vi "Find_Mid_Value.vi"() -> ()   [LabVIEW 2020]
uses:
  <vilib>/DAQmx/read.llb/DAQmx Read (Analog DBL 1Chan 1Samp).vi
  <vilib>/Analysis/baseanly.llb/Mean (DBL).vi
  <vilib>/DAQmx/create/channels.llb/DAQmx Create Channel (AI-Voltage-Basic).vi
  <vilib>/DAQmx/configure/timing.llb/DAQmx Timing (Sample Clock).vi
  <vilib>/DAQmx/miscellaneous.llb/DAQmx Fill In Error Info.vi
  <vilib>/Analysis/NI_AALBase.lvlib
panel:
  out "mean":dbl format="%0.2f"
  out "Final Array":dbl[][](array[numeric])
  out "Initialized Array":dbl[][](array[numeric])
  out "Temperature Array":dbl[][](array[numeric])
  out "error out":errorcluster
  in  "Columns":u8
  in  "Rows":u8
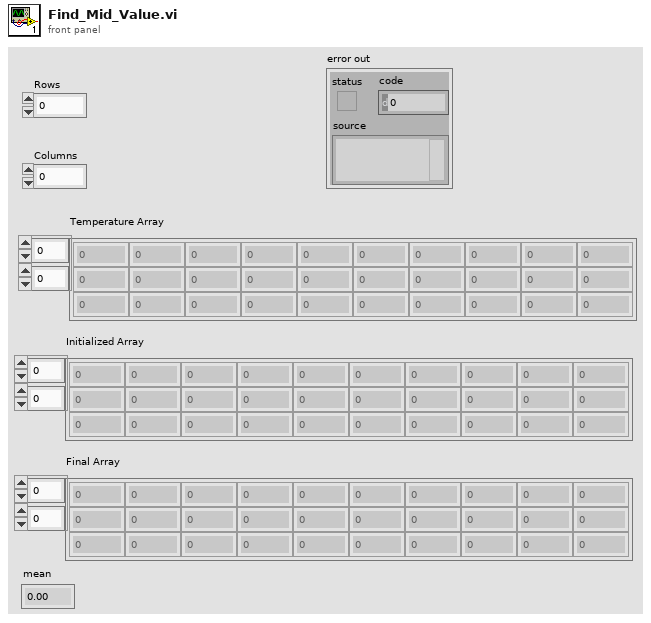
[diagram p1: front panel]
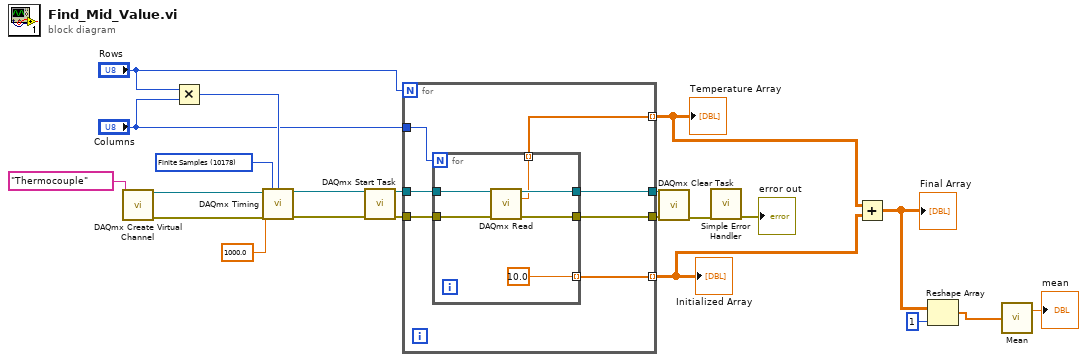
[diagram p0: block diagram]
diagram:
  w18 = 10178 items=["Finite Samples"=10178, "Continuous Samples"=10123, "Hardware Timed Single Point"=12522] ("sample mode")
  n1 = call-poly <vilib>:"DAQmx Create Virtual Channel.vi"("physical channels"=tag "Thermocouple") -> ("task out"=w20:refnum<k21>, "error out"=w21:errorcluster)  [unwired: 13 in]
  n2 = Multiply(x="Rows", y="Columns") -> (x*y=w17:u8)
  n3 = call-poly <vilib>:"DAQmx Timing.vi"("task/channels in"=w20, "sample mode"=w18, "samples per channel"=w17, "rate"=1000.0, "error in"=w21) -> ("task out"=w16:refnum<k21>, "error out"=w15:errorcluster)  [unwired: 9 in]
  n4 = call <vilib>:"DAQmx Start Task.vi"("task/channels in"=w16, "error in"=w15) -> ("task out"=w13:refnum<k21>, "error out"=w14:errorcluster)  [unwired: 12 in]
  n5 = for {
    N: "Rows" -> [_]
    tunnel: "Columns" -> [w25]
    tunnel: w13 -> [w28]
    tunnel: [w27] -> w12
    tunnel: w14 -> [w29]
    tunnel: [w26] -> w11
    tunnel: [w24] -> w6 mode=indexing
    tunnel: [w23] -> w5 mode=indexing
    n6 = for {
      N: w25 -> [_]
      tunnel: w28 -> [w34]
      tunnel: [w33] -> w27
      tunnel: w29 -> [w35]
      tunnel: [w32] -> w26
      tunnel: [w31] -> w24 mode=indexing
      tunnel: [10.0] -> w23 mode=indexing
      n7 = call-poly <vilib>:"DAQmx Read.vi"("task/channels in"=w34, "error in"=w35) -> ("task out"=w33:refnum<k21>, "data"=w31:dbl, "error out"=w32:errorcluster)  [unwired: 11 in]
    }
  }
  "Temperature Array" <- w6
  "Initialized Array" <- w5
  n8 = call <vilib>:"DAQmx Clear Task.vi"("task in"=w12, "error in"=w11) -> ("error out"=w10:errorcluster)  [unwired: 13 in]
  n9 = call <vilib>:"Simple Error Handler.vi"("error in (no error)"=w10) -> ("error out"=→"error out":errorcluster)  [unwired: 4 in, 4 out]
  n10 = Add(x=w6, y=w5) -> (x+y=w3:dbl[][])
  "Final Array" <- w3
  n11 = Reshape Array(w3, 1 ("dimension size")) -> (w1:dbl[])
  n12 = call-poly <vilib>:"Mean.vi"("X"=w1) -> ("mean"=→"mean":dbl)  [unwired: 1 out]
